vi "RxBfrPkt - Add Packet.vi"(7 "Ext Buffer?":bool, 8 "error in (no error)":errorcluster, 9 "New Packet ID":i32, 10 "New Packet Name":string, 11 "Item Ref in":T1=18446744073709551615 format="%.0x") -> (0 "error out":errorcluster, 2 "New Packet Ref":T1=18446744073709551615 format="%.0x", 3 "Item Ref Out":T1=18446744073709551615 format="%.0x")   [LabVIEW 2016, in "UDP-Custom-Device System Explorer.lvlib"]
uses:
  UDP-Custom-Device System Explorer.lvlib
  <vilib>/NI Veristand/Custom Device API/Custom Device Item Ref.ctl
  Shared/Constants.vi
  Property Accessors/Shared Section Accessors.lvlib
  <vilib>/NI VeriStand/Custom Device API/Custom Device API.lvlib
  Property Accessors/Shared Packet Accessors.lvlib
  Shared/UDP-Custom-Device Shared.lvlib
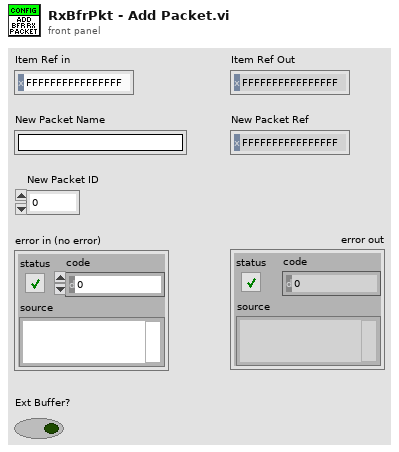
[diagram p1: front panel]
types:
  T1 = typedef "Custom Device API.lvlib/Custom Device Item Ref.ctl" = u64
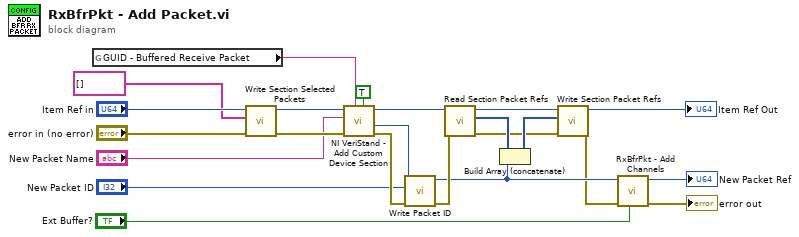
[diagram p0: block diagram]
diagram:
  n1 = global read "Constants.vi" "GUID - Buffered Receive Packet"() -> (w6:string)
  n2 = call "Write Section Selected Packets.vi"("error in (no error)"="error in (no error)", "Selected Packets"=string[] [] ("Value"), "Node Ptr"="Item Ref in") -> ("error out"=w15:errorcluster, "Node Ptr out"=w14:T1)  [unwired: 7 in]
  n3 = call <vilib>:"NI VeriStand - Add Custom Device Section.vi"("Highlight? (F)"=TRUE, "GUID (Default Section)"=w6, "error in (no error)"=w15, "Section Name"="New Packet Name", "Parent Ref in"=w14) -> ("error out"=w23:errorcluster, "Section Ptr"=w22:T1, "Parent Ref out"=w21:T1)  [unwired: 3 in, 1 out]
  n4 = call "Write Packet ID.vi"("error in (no error)"=w23, "Packet ID"="New Packet ID", "Node Ptr"=w22) -> ("error out"=w16:errorcluster, "Node Ptr out"=w5:T1)  [unwired: 7 in]
  n5 = call "Read Section Packet Refs.vi"("error in (no error)"=w16, "Node Ptr"=w21) -> ("error out"=w17:errorcluster, "Dependent Node Refs"=w19:T1[], "Node Ptr out"=w20:T1)  [unwired: 7 in]
  n6 = Build Array (concatenate)(w19, w5) -> (w18:T1[])
  n7 = call "Write Section Packet Refs.vi"("error in (no error)"=w17, "Dependent Node Refs"=w18, "Node Ptr"=w20) -> ("error out"=w3:errorcluster, "Node Ptr out"=→"Item Ref Out":T1)  [unwired: 7 in]
  n8 = call "RxBfrPkt - Add Channels.vi"("Ext Buffer?"="Ext Buffer?", "error in (no error)"=w3, "Node Ptr"=w5) -> ("error out"=→"error out":errorcluster, "Node Ptr out"=→"New Packet Ref":T1)  [unwired: 7 in]
